vi "Process VIA.vi"(8 "error in (no error)":errorcluster, 10 "Raw VIA":string, 11 "RP2040Target in":refnum<class "RP2040Target.lvclass">) -> (0 "error out":errorcluster, 2 "VIA":string, 3 "RP2040Target out":refnum<class "RP2040Target.lvclass">)   [LabVIEW 2020, in "RP2040.lvlib" / "RP2040Target.lvclass"]
uses:
  RP2040Target.lvclass
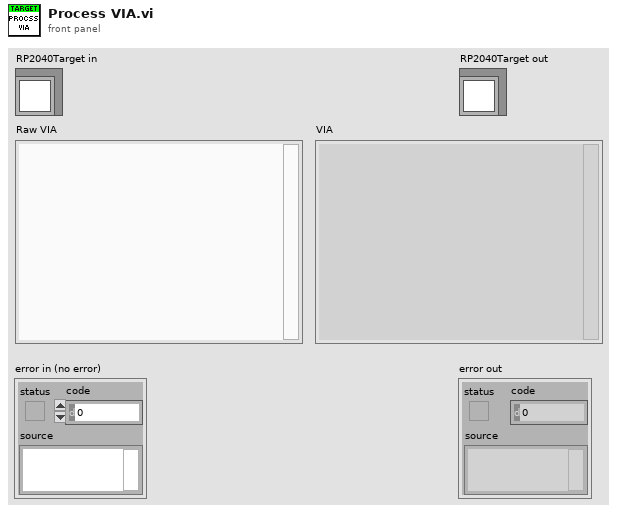
[diagram p1: front panel]
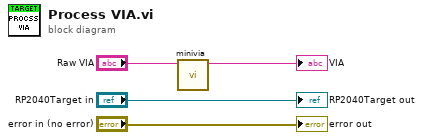
[diagram p0: block diagram]
diagram:
  n1 = call "minivia.vi"("VIA"="Raw VIA") -> ("Minified"=→"VIA":string)  [unwired: 10 in]
  "error out" <- "error in (no error)"
  "RP2040Target out" <- "RP2040Target in"
